vi "Psi and Delta Mapping_V2.3_RCE P=0_A_45_stokes vector.vi"() -> ()   [LabVIEW 2022 SP3]
uses:
  <vilib>/Math Plots/3D Math Plots/3D Surface/3D Surface XCtrl/3D Surface.xctl
  <vilib>/Analysis/baseanly.llb/Real A x B.vi
  <vilib>/Analysis/baseanly.llb/A x Vector.vi
  <vilib>/Utility/file.llb/Read Delimited Spreadsheet (I64).vi
  <vilib>/Analysis/baseanly.llb/Real Inverse Matrix.vi
  <vilib>/Math Plots/3D Math Plots/3D Surface/3D Surface Datatype/Public/Plot Helper (Matrix).vi
  <vilib>/Utility/file.llb/Write Delimited Spreadsheet (DBL).vi
  <vilib>/Utility/file.llb/Read Delimited Spreadsheet (DBL).vi
  <vilib>/Math Plots/3D Math Plots/3D Surface/3D Surface Datatype/3D Surface Datatype.lvclass
  <vilib>/Analysis/NI_AALBase.lvlib
panel:
  out "transposed array":dbl[][](array[numeric])
  out "x+1":i8
  in  "Tab Control":enum32{"Psi & Delta Mapping"}(tab)
  out "Drag the ROI":i64[][](graph)
  out "Location of ROI":cluster{dbl[], dbl[]}(graph)
  in  "Sampling Range (nm):":string(combo)="5"
  out "Intensity Graph 2":i64[][](graph)
  in  "Distance":dbl(slide)=1.525974025974026 scale=0.0..2.5
  in  "Map BMP File":bool
  in  "Map ASCII File":bool
  out "Psi":dbl[][](graph)
  out "Delta":dbl[][](graph)
  out "concatenated string":string
  out "concatenated string 2":string
  out "Psi Surface":refnum<class "3D Plot Datatype.lvclass">[](xcontrol)
  in  "Start (nm) :":i16=400
  in  "End (nm) :":i16=700
  in  "Save the files ?":bool
  in  "Choose an arbitrary file in the angle of incidence folder :":path
  out "Files currently reading":string
  out "Seconds":dbl
  out "Minutes":dbl
  out "Hours":dbl
  out "Delta Surface":refnum<class "3D Plot Datatype.lvclass">[](xcontrol)
  out "uniformity":cluster{i32[], dbl[]}(graph)
  out "ALL":cluster{dbl[], dbl[]}[](graph)
  in  "SE BMP & Txt File":bool
  out "Pixels :":i32(slide) scale=0.0..100.0
  in  "Psi data base":path=path "C:/Users/王家麟/Desktop/_Data/Model generate/SiO2_300nm_psi.txt"
  in  "Model index AOI25=1 ~AOI75=11":i32=4
  in  "delta data base":path=path "C:/Users/王家麟/Desktop/_Data/Model generate/SiO2_300nm_delta.txt"
  in  "Angle of Incidence :":string(combo)="55"
  out "PSI":dbl
  out "DELTA":dbl
  out "PPSI":dbl
  out "PDELTA":dbl
  out "B2":dbl
  out "a4":dbl
  out "B4":dbl
  out "XY Graph":cluster{dbl[], dbl[]}[](graph)
  in  "Psi data base 2":path=path "C:/Users/王家麟/Desktop/12.29_2D data/AOI_40_SE data_Ins_polar_285.5nm.txt"
  in  "Ins loaded":bool
  # "Wavelength Setting :"
  # "YES"
  # "NO"
  # "%"
  # "Ins index"
  # "Time spent :"
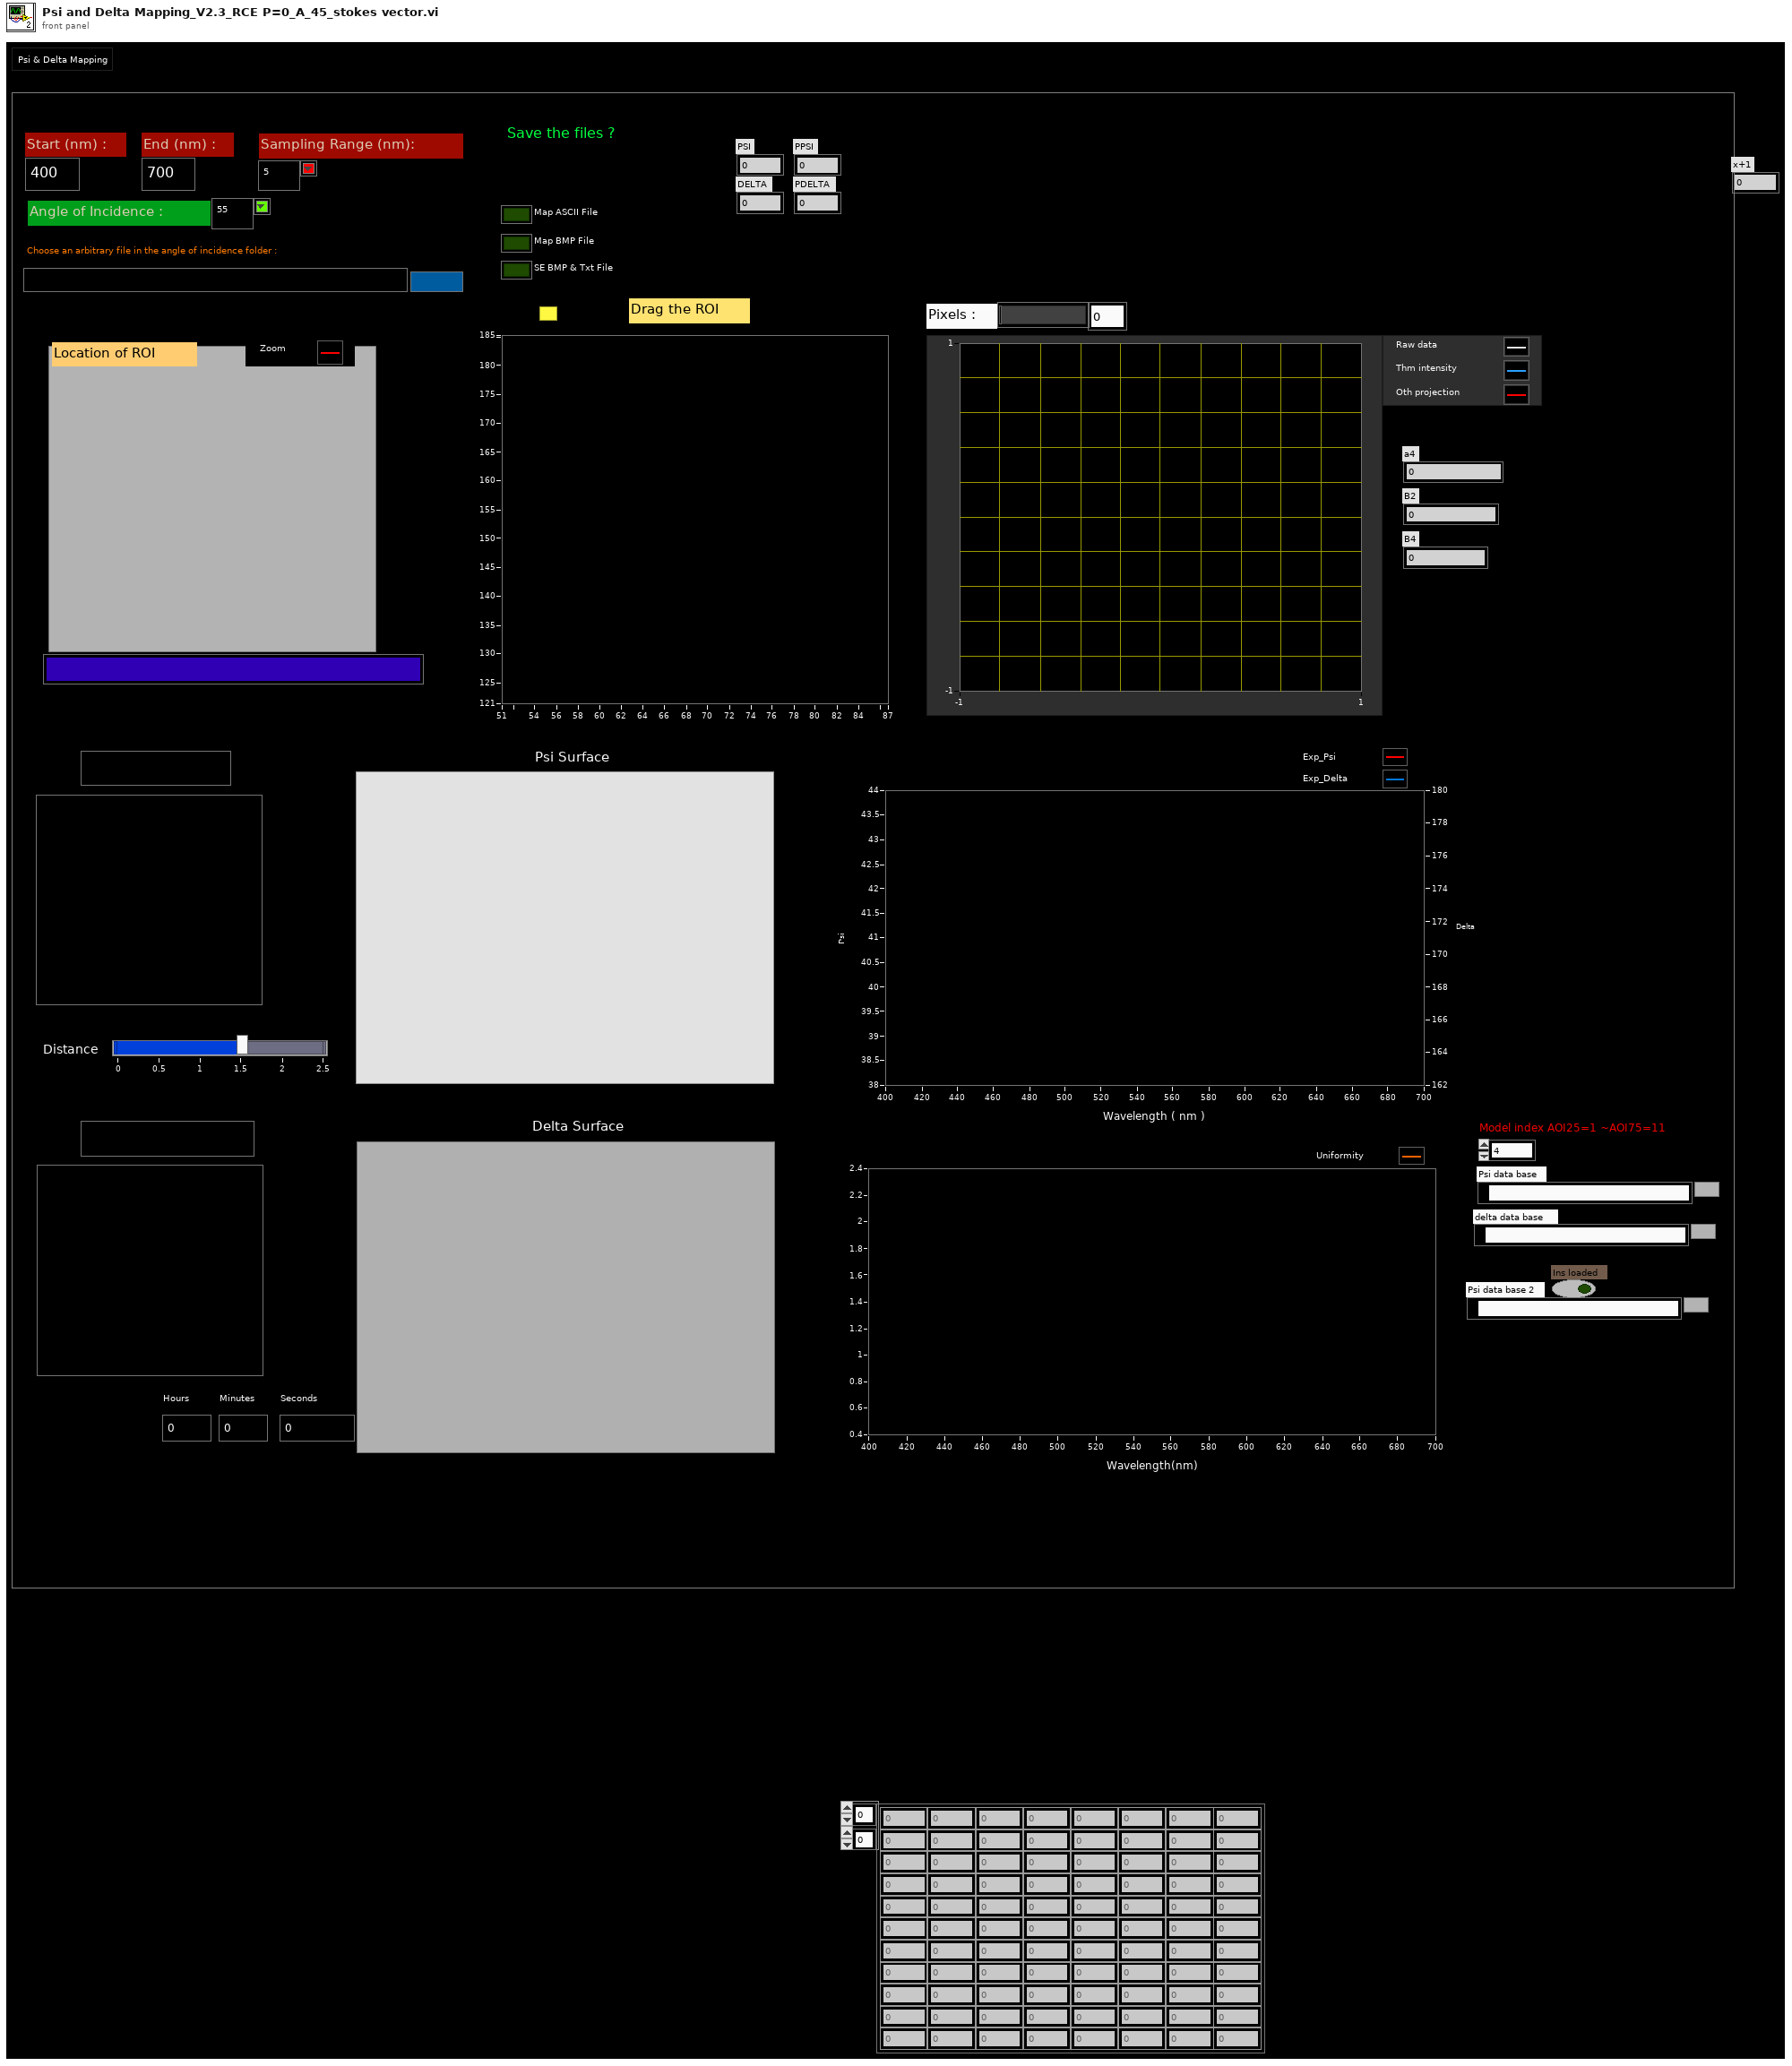
[diagram p1: front panel]
types:
  T1 = typedef "NI_Matrix.lvlib/RealMatrix.ctl" = dbl[][]
  T2 = typedef "imagedata.ctl" = cluster{"image type":i32, "image depth":i32, "image":u8[], "mask":u8[], "colors":u32[], "Rectangle":cluster{"left":i16, "top":i16, "right":i16, "bottom":i16}}
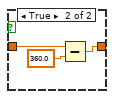
[diagram p3: hidden frame]
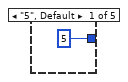
[diagram p4: hidden frame]
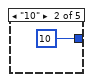
[diagram p5: hidden frame]
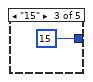
[diagram p6: hidden frame]
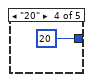
[diagram p7: hidden frame]
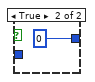
[diagram p8: hidden frame]
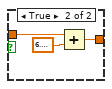
[diagram p9: hidden frame]
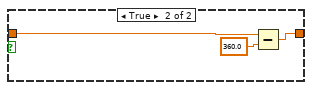
[diagram p12: hidden frame]
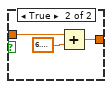
[diagram p13: hidden frame]
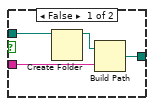
[diagram p19: hidden frame]
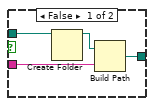
[diagram p20: hidden frame]
diagram:
  (unwired) TRUE
  (unwired) TRUE
  n1 = flat-sequence {
    tunnel: [w86] -> w8
    tunnel: [w84] -> w7
    tunnel: [w83] -> w6
    tunnel: [w21] -> w5
    tunnel: [w10] -> w4
    tunnel: [w9] -> w3
    tunnel: [w22] -> w2
    tunnel: [w20] -> w1
    tunnel: w8 -> [w681]
    tunnel: w7 -> [w680]
    tunnel: w6 -> [w679]
    tunnel: w5 -> [w678]
    tunnel: w4 -> [w677]
    tunnel: w3 -> [w676]
    tunnel: w2 -> [w675]
    tunnel: w1 -> [w674]
    frame #0 {
      w18 = u32 0 ("Plot.Y Scale Index")
      w17 = u32 1 ("Plot.Y Scale Index")
      n2 = property on="ALL" class="XYGraph (strict)"("Active Plot"=u32 0, "Plot.YScaleIdx"=w17, "Active Plot"=u32 1, "Plot.YScaleIdx"=w18, "Active Plot"=u32 2, "Plot.YScaleIdx"=w17, "Active Plot"=u32 3, "Plot.YScaleIdx"=w18, "Active Plot"=u32 4, "Plot.YScaleIdx"=w17, "Active Plot"=u32 5, "Plot.YScaleIdx"=w18, "Active Plot"=u32 6, "Plot.YScaleIdx"=w17, "Active Plot"=u32 7, "Plot.YScaleIdx"=w18) -> ()  [unwired: 2 in, 2 out]
      n3 = flat-sequence {
        tunnel: [w140] -> w62
        tunnel: "Choose an arbitrary file in the angle of incidence folder :" -> [w141]
        tunnel: w62 -> [w145]
        tunnel: [w145] -> w61
        tunnel: w61 -> [w148]
        tunnel: [w149] -> w60
        tunnel: [w150] -> w59
        tunnel: [w151] -> w58
        tunnel: [w152] -> w57
        tunnel: [w162] -> w63
        tunnel: [w163] -> w64
        tunnel: w60 -> [w158]
        tunnel: w59 -> [w163]
        tunnel: w58 -> [w159]
        tunnel: w57 -> [w162]
        tunnel: [w157] -> w56
        tunnel: [w156] -> w55
        frame #0 {
          n4 = call-poly <vilib>:"Read Delimited Spreadsheet.vi"("file path (dialog if empty)"=w141) -> ("all rows"=w140:i64[][])  [unwired: 9 in, 5 out]
        }
        frame #1 {
          w142 = 0 ("index")
          n5 = Array Size(array=w145) -> (size(s)=w147:i32[])
          n6 = Index Array(array=w147, index=w142) -> (element=w143:i32)
          n7 = Index Array(array=w147, index=1) -> (element=w144:i32)
          n8 = property on="Intensity Graph 2" class="IntGraph (strict)"("XScale.Maximum"=w143, "XScale.Minimum"=w142) -> ()  [unwired: 2 in, 2 out]
          n9 = property on="Intensity Graph 2" class="IntGraph (strict)"("YScale.Maximum"=w144, "YScale.Minimum"=w142) -> ()  [unwired: 2 in, 2 out]
        }
        frame #2 {
          "Drag the ROI" <- w148
        }
        frame #3 {
          n10 = property on="Drag the ROI" class="IntGraph (strict)"() -> ("XScale.Maximum"=w149:dbl, "XScale.Minimum"=w150:dbl)  [unwired: 2 in, 2 out]
          n11 = property on="Drag the ROI" class="IntGraph (strict)"() -> ("YScale.Maximum"=w151:dbl, "YScale.Minimum"=w152:dbl)  [unwired: 2 in, 2 out]
          n12 = Build Array(w150, w150, w149, w149, w150) -> (w155:dbl[])
          n13 = Build Array(w152, w151, w151, w152, w152) -> (w154:dbl[])
          n14 = Bundle(w155, w154) -> (→"Location of ROI":cluster{dbl[], dbl[]})  [unwired: 1 in]
        }
        frame #4 {
          n15 = Subtract(x=w158, y=w163) -> (x-y=w161:dbl)
          n16 = Subtract(x=w159, y=w162) -> (x-y=w160:dbl)
          n17 = Increment(x=w161) -> (x+1=w156:dbl)
          n18 = Increment(x=w160) -> (x+1=w157:dbl)
        }
      }
      n19 = case shown="\"25\"" "Sampling Range (nm):" {
        tunnel: [i8 5 i8 10 i8 15 i8 20 i8 25] -> w14
        frame "5", Default {
        }
        frame "10" {
        }
        frame "15" {
        }
        frame "20" {
        }
        frame "25" {
        }
      }
      n20 = Subtract(x="End (nm) :", y="Start (nm) :") -> (x-y=w70:i16)
      n21 = Divide(x=w70, y=w14) -> (x/y=w71:dbl)
      n22 = Strip Path(path="Choose an arbitrary file in the angle of incidence folder :") -> (stripped path=w28:path)  [unwired: 1 out]
      n23 = Increment(x=w71) -> (x+1=w66:dbl)
      "x+1" <- w66
      n24 = Strip Path(path=w28) -> (stripped path=w29:path)  [unwired: 1 out]
      n25 = Path To String(path=w29) -> (string=w87:string)
      n26 = for {
        N: w66 -> [_]
        tunnel: w28 -> [w172]
        tunnel: w87 -> [w201]
        tunnel: [w193] -> w73 mode=indexing
        tunnel: [w189] -> w21 mode=indexing
        tunnel: [w187] -> w74 mode=indexing
        tunnel: [w185] -> w12 mode=indexing
        tunnel: [w173] -> w84
        tunnel: [w182] -> w83
        tunnel: w14 -> [w180]
        tunnel: w56 -> [w179]
        tunnel: w55 -> [w178]
        tunnel: w63 -> [w177]
        tunnel: w64 -> [w176]
        tunnel: [w169] -> w19 mode=indexing
        i -> [w212]
        n27 = flat-sequence {
          tunnel: w212 -> [w235]
          tunnel: [w228] -> w211
          tunnel: [w227] -> w210
          tunnel: [w226] -> w209
          tunnel: [w225] -> w208
          tunnel: [w224] -> w207
          tunnel: [w223] -> w205
          tunnel: w172 -> [w213]
          tunnel: w201 -> [w222]
          tunnel: [w220] -> w190
          tunnel: [w219] -> w186
          tunnel: w180 -> [w218]
          tunnel: w179 -> [w217]
          tunnel: w178 -> [w216]
          tunnel: w177 -> [w215]
          tunnel: w176 -> [w214]
          tunnel: [w213] -> w175
          tunnel: w211 -> [w352]
          tunnel: w210 -> [w351]
          tunnel: w209 -> [w350]
          tunnel: w208 -> [w359]
          tunnel: w207 -> [w358]
          tunnel: [w356] -> w206
          tunnel: w205 -> [w356]
          tunnel: [w355] -> w202
          tunnel: [w354] -> w200
          tunnel: [w353] -> w199
          tunnel: [w346] -> w191
          tunnel: w190 -> [w346]
          tunnel: w186 -> [w342]
          tunnel: [w329] -> w184
          tunnel: w175 -> [w355]
          tunnel: [w318] -> w171
          tunnel: w206 -> [w550]
          tunnel: ["Save the files ?"] -> w204
          tunnel: [w545] -> w203
          tunnel: w202 -> [w545]
          tunnel: w200 -> [w544]
          tunnel: w199 -> [w543]
          tunnel: [w541] -> w198
          tunnel: [w542] -> w197
          tunnel: [w527] -> w196
          tunnel: [w531] -> w195
          tunnel: [w529] -> w194
          tunnel: [w528] -> w192
          tunnel: w191 -> [w528]
          tunnel: [w519] -> w188
          tunnel: w184 -> [w518]
          tunnel: [w518] -> w183
          tunnel: ["Save the files ?"] -> w182
          tunnel: ["Map BMP File"] -> w181
          tunnel: w171 -> [w514]
          tunnel: [w514] -> w170
          tunnel: w194 -> [w558]
          tunnel: w195 -> [w559]
          tunnel: w196 -> [w560]
          tunnel: w197 -> [w561]
          tunnel: w198 -> [w562]
          tunnel: w203 -> [w563]
          tunnel: w204 -> [w564]
          tunnel: [w558] -> w193
          tunnel: [w557] -> w189
          tunnel: w192 -> [w557]
          tunnel: [w556] -> w187
          tunnel: w188 -> [w556]
          tunnel: [w555] -> w185
          tunnel: w183 -> [w555]
          tunnel: [w554] -> w174
          tunnel: w181 -> [w553]
          tunnel: w170 -> [w552]
          tunnel: [w552] -> w169
          frame #0 {
            n28 = Multiply(x=w235, y=w218) -> (x*y=w237:i32)
            n29 = local read "Start (nm) :"() -> (w236:i16)
            n30 = Add(x=w236, y=w237) -> (x+y=w220:i32)
            n31 = Number To Decimal String(number=w220) -> (decimal integer string=w223:string)  [unwired: 1 in]
            n32 = Concatenate Strings(w222, "\\" ("string"), w223, "nm\\" ("string")) -> (w233:string)
            n33 = for {
              N: i8 15 -> [_]
              tunnel: w233 -> [w260]
              tunnel: w223 -> [w259]
              tunnel: [w258] -> w228 mode=indexing
              tunnel: [w256] -> w225
              tunnel: [w255] -> w224
              tunnel: [w257] -> w219 mode=indexing
              tunnel: w217 -> [w254]
              tunnel: w216 -> [w253]
              tunnel: w215 -> [w252]
              tunnel: w214 -> [w251]
              i -> [w263]
              n34 = Increment(x=w263) -> (x+1=w262:i32)
              n35 = Number To Decimal String(number=w262) -> (decimal integer string=w266:string)  [unwired: 1 in]
              n36 = Concatenate Strings(w260, w259, " (" ("string"), w266, ").asc" ("string")) -> (w265:string)
              n37 = String To Path(string=w265) -> (path=w250:path)
              n38 = flat-sequence {
                tunnel: w250 -> [w275]
                tunnel: w251 -> [w276]
                tunnel: w252 -> [w277]
                tunnel: w253 -> [w278]
                tunnel: w254 -> [w279]
                tunnel: [w279] -> w242
                tunnel: [w278] -> w241
                tunnel: [w277] -> w240
                tunnel: [w276] -> w239
                tunnel: [w267] -> w238
                tunnel: [w295] -> w249
                tunnel: [w289] -> w248
                tunnel: [w288] -> w247
                tunnel: [w292] -> w246
                tunnel: [w288] -> w245
                tunnel: [w290] -> w244
                tunnel: [w291] -> w243
                tunnel: w238 -> [w280]
                tunnel: w239 -> [w284]
                tunnel: w240 -> [w285]
                tunnel: w241 -> [w286]
                tunnel: w242 -> [w287]
                tunnel: [w301] -> w255
                tunnel: [w302] -> w256
                tunnel: [w303] -> w257
                tunnel: [w296] -> w258
                tunnel: w249 -> [w303]
                tunnel: w248 -> [w302]
                tunnel: w247 -> [w301]
                tunnel: w246 -> [w300]
                tunnel: w245 -> [w299]
                tunnel: w244 -> [w298]
                tunnel: w243 -> [w297]
                frame #0 {
                  n39 = call-poly <vilib>:"Read Delimited Spreadsheet.vi"("file path (dialog if empty)"=w275) -> ("new file path (Not A Path if cancelled)"=w274:path, "all rows"=w267:i64[][])  [unwired: 9 in, 4 out]
                  "Intensity Graph 2" <- w267
                  n40 = Strip Path(path=w274) -> (stripped path=w273:path, name=w270:string)
                  n41 = Strip Path(path=w273) -> (name=w272:string)  [unwired: 1 out]
                  n42 = Concatenate Strings("Files currently reading : " ("string"), w272, "\\" ("string"), w270) -> (→"Files currently reading":string)
                }
                frame #1 {
                  w291 = 75 ("Dark counts")
                  n43 = Array Subset(array=w280, index (row)=w284, length (row)=w286, index (col)=w285, length (col)=w287) -> (w290:i64[][])
                  n44 = local write "Drag the ROI"(w280) -> ()
                  n45 = Add Array Elements(numeric array=w290) -> (sum=w294:i64)
                  n46 = Array Size(array=w290) -> (size(s)=w283:i32[])
                  n47 = Index Array(array=w283, index=1) -> (element=w289:i32)
                  n48 = Index Array(array=w283, index=0) -> (element=w288:i32)
                  n49 = Multiply(x=w289, y=w288) -> (x*y=w292:i32)
                  n50 = Multiply(x=w292, y=w291) -> (x*y=w293:i32)
                  n51 = Subtract(x=w294, y=w293) -> (x-y=w295:i64)
                }
                frame #2 {
                  n52 = for {
                    N: w300 -> [_]
                    tunnel: w299 -> [w312]
                    tunnel: w298 -> [w304]
                    tunnel: [w307] -> w296 mode=indexing
                    tunnel: w297 -> [w306]
                    i -> [w313]
                    n53 = Quotient & Remainder(x=w313, y=w312) -> (x-y*floor(x/y)=w311:i32, floor(x/y)=w310:i32)
                    n54 = Index Array(array=w304, index (row)=w311, index (col)=w310) -> (element=w305:i64)
                    n55 = Subtract(x=w305, y=w306) -> (x-y=w308:i64)
                    n56 = Less Than 0?(x=w308) -> (x < 0?=w309:bool)
                    n57 = case shown="False" w309 {
                      tunnel: [w314 i8 0] -> w307
                      tunnel: w308 -> [w314 _]
                      frame False {
                      }
                      frame True {
                      }
                    }
                  }
                }
              }
            }
            n58 = Array Size(array=w228) -> (size(s)=w229:i32[])
            n59 = Index Array(array=w229, index=1) -> (element=w226:i32)
            n60 = Index Array(array=w229, index=0) -> (element=w227:i32)
          }
          frame #1 {
            w357 = 0.0
            n61 = property on="Delta" class="IntGraph (strict)"("YScale.Maximum"=w359, "YScale.Minimum"=w357) -> ()  [unwired: 2 in, 2 out]
            n62 = for {
              N: i8 15 -> [_]
              tunnel: [w383] -> w340 mode=indexing
              tunnel: [w382] -> w341 mode=indexing
              i -> [w386]
              n63 = Increment(x=w386) -> (x+1=w385:i32)
              n64 = Multiply(x=24.0, y=w385) -> (x*y=w382:dbl)
              n65 = expression code="(x/180.0)*pi" "degrees to radians"(w382) -> (w381:dbl)
              n66 = formula code="float c1,c2,c3,c4;\nc1=1;\nc2=sin(2*C);\nc3=cos(4*C);\nc4=sin(4*C);"("C"=w381) -> ("c2"=w380:dbl, "c3"=w379:dbl, "c4"=w378:dbl, "c1"=w377:dbl)
              n67 = Build Array(w377, w380, w379, w378) -> (w383:dbl[])
            }
            n68 = property on="Psi" class="IntGraph (strict)"("YScale.Maximum"=w359, "YScale.Minimum"=w357) -> ()  [unwired: 2 in, 2 out]
            n69 = property on="Psi" class="IntGraph (strict)"("XScale.Maximum"=w358, "XScale.Minimum"=w357) -> ()  [unwired: 2 in, 2 out]
            n70 = property on="Delta" class="IntGraph (strict)"("XScale.Maximum"=w358, "XScale.Minimum"=w357) -> ()  [unwired: 2 in, 2 out]
            n71 = Transpose 2D Array(2D array=w340) -> (transposed array=w339:dbl[][])
            n72 = for {
              N: w350 -> [w458]
              tunnel: w352 -> [w464]
              tunnel: w351 -> [w461]
              tunnel: [w387] -> w349 mode=indexing
              tunnel: [w443] -> w348 mode=indexing
              tunnel: w340 -> [w451]
              tunnel: w341 -> [w435]
              i -> [w460]
              n73 = Transpose 2D Array(2D array=w451) -> (transposed array=w450:dbl[][])
              n74 = call-poly <vilib>:"A x B.vi"("B"=w451, "A"=w450) -> ("A x B"=w454:T1)  [unwired: 1 out]
              n75 = Increment(x=w460) -> (x+1=w459:i32)
              n76 = Array Subset(array=w464, index (col)=w460, length (col)=1 ("length")) -> (w462:i64[][])  [unwired: 2 in]
              n77 = Divide(x=w459, y=w458) -> (x/y=w457:dbl)
              n78 = call-poly <vilib>:"Inverse Matrix.vi"("Input Matrix"=w454) -> ("Inverse Matrix"=w453:T1)  [unwired: 1 in, 1 out]
              n79 = Reshape Array(w462, w461) -> (w422:i64[])
              n80 = call-poly <vilib>:"A x B.vi"("B"=w450, "A"=w453) -> ("A x B"=w452:T1)  [unwired: 1 out]
              n81 = Array Max & Min(array=w422) -> (max value=w423:i64)  [unwired: 3 out]
              n82 = Multiply(x=i8 100, y=w457) -> (x*y=→"Pixels :":dbl)
              n83 = Divide(x=w422, y=w423) -> (x/y=w421:dbl[])
              n84 = call-poly <vilib>:"A x B.vi"("Vector"=w422, "A"=w452) -> ("A x Vector"=w449:dbl[])  [unwired: 1 out]
              n85 = call-poly <vilib>:"A x B.vi"("Vector"=w449, "A"=w451) -> ("A x Vector"=w416:dbl[])  [unwired: 1 out]
              n86 = Index Array(array=w449, index #1=0 ("index"), index #2=1 ("index"), index #3=2 ("index"), index #4=3 ("index")) -> (element #1=w425:dbl, element #2=w434:dbl, element #3=w444:dbl, element #4=w433:dbl)
              n87 = Array Max & Min(array=w416) -> (max value=w417:dbl)  [unwired: 3 out]
              n88 = formula code="float psi, delta ;\n\npsi = 0.5*atan(sqrt((0.5*B2)**2+\n                           (B4)**2)/(-a4)) ;\ndelta = atan(0.5*B2/B4) ;\nx=sign(B2);\ny=sign(B4);"("B2"=w434, "a4"=w444, "B4"=w433, "r"=w425) -> ("psi"=w441:dbl, "delta"=w427:dbl, "x"=w426:dbl, "y"=w428:dbl)
              n89 = Divide(x=w416, y=w417) -> (x/y=w415:dbl[])
              n90 = Greater Than 0?(x=w426) -> (x > 0?=w432:bool)
              n91 = Greater Than 0?(x=w428) -> (x > 0?=w430:bool)
              n92 = Less Than 0?(x=w441) -> (x < 0?=w442:bool)
              n93 = And(x=w432, y=w430) -> (x .and. y?=w431:bool)
              n94 = case shown="True" w442 {
                tunnel: w441 -> [w494 w497]
                tunnel: [w494 w496] -> w440
                frame False {
                }
                frame True {
                  n95 = Add(x=w497, y=1.5707963267948966) -> (x+y=w496:dbl)
                }
              }
              n96 = case shown="False" w431 {
                tunnel: w427 -> [w486 w493]
                tunnel: [w484 w493] -> w429
                tunnel: w426 -> [w485 _]
                tunnel: w430 -> [w481 _]
                frame False {
                  n97 = Less Than 0?(x=w485) -> (x < 0?=w483:bool)
                  n98 = And(x=w481, y=w483) -> (x .and. y?=w482:bool)
                  n99 = case shown="False" w482 {
                    tunnel: w486 -> [w487 w491]
                    tunnel: [w488 w490] -> w484
                    frame False {
                      n100 = Add(x=w487, y=3.141592653589793) -> (x+y=w488:dbl)
                    }
                    frame True {
                      n101 = Add(x=w491, y=6.283185307179586) -> (x+y=w490:dbl)
                    }
                  }
                }
                frame True {
                }
              }
              n102 = expression code="(x/pi)*180.0" "radians to degrees"(w440) -> (w443:dbl)
              "PPSI" <- w443
              n103 = expression code="(x/pi)*180.0" "radians to degrees"(w429) -> (w388:dbl)
              n104 = for {
                tunnel: w425 -> [w503]
                tunnel: [w502] -> w419 mode=indexing
                tunnel: w435 -> [w501] mode=indexing
                tunnel: w440 -> [w499]
                tunnel: w429 -> [w500]
                tunnel: [w498] -> w424 mode=indexing
                n105 = expression code="(x/180.0)*pi" "degrees to radians"(w501) -> (w498:dbl)
                n106 = formula code="float S1,S2 ,S3;\n\nS1 = - cos(2*a);\nS2 =  sin(2*a)*cos(b);\nS3 = -sin(2*a)*sin(b);\nI = r * (1+0.577*S1*cos(4*C)\n           -S3*sin(2*C)\n            +0.5*S2*sin(4*C)) ;"("r"=w503, "a"=w499, "b"=w500, "C"=w498) -> ("I"=w502:dbl)
              }
              n107 = Greater?(x=w388, y=360.0) -> (0:w390:bool)
              n108 = case shown="False" w390 {
                tunnel: w388 -> [w465 w467]
                tunnel: [w465 w466] -> w387
                frame False {
                }
                frame True {
                  n109 = Subtract(x=w467, y=360.0) -> (x-y=w466:dbl)
                }
              }
              "PDELTA" <- w387
              n110 = for {
                tunnel: w421 -> [w480] mode=indexing
                tunnel: w424 -> [w479] mode=indexing
                tunnel: [w478] -> w412 mode=indexing
                tunnel: [w477] -> w400 mode=indexing
                n111 = formula code="float x,y;\nx=I*cos(p);\ny=I*sin(p);"("I"=w480, "p"=w479) -> ("x"=w478:dbl, "y"=w477:dbl)
              }
              n112 = Array Max & Min(array=w419) -> (max value=w420:dbl)  [unwired: 3 out]
              n113 = for {
                tunnel: w415 -> [w472] mode=indexing
                tunnel: w424 -> [w471] mode=indexing
                tunnel: [w470] -> w404 mode=indexing
                tunnel: [w469] -> w392 mode=indexing
                n114 = formula code="float x,y;\nx=I*cos(p);\ny=I*sin(p);"("I"=w472, "p"=w471) -> ("x"=w470:dbl, "y"=w469:dbl)
              }
              n115 = Divide(x=w419, y=w420) -> (x/y=w418:dbl[])
              n116 = for {
                tunnel: w418 -> [w476] mode=indexing
                tunnel: w424 -> [w475] mode=indexing
                tunnel: [w474] -> w408 mode=indexing
                tunnel: [w473] -> w396 mode=indexing
                n117 = formula code="float x,y;\nx=I*cos(p);\ny=I*sin(p);"("I"=w476, "p"=w475) -> ("x"=w474:dbl, "y"=w473:dbl)
              }
              n118 = Index Array(array=w412, index=0) -> (element=w413:dbl)
              n119 = Index Array(array=w400, index=0) -> (element=w401:dbl)
              n120 = Index Array(array=w404, index=0) -> (element=w405:dbl)
              n121 = Index Array(array=w392, index=0) -> (element=w393:dbl)
              n122 = Build Array (concatenate)(w412, w413) -> (w411:dbl[])
              n123 = Build Array (concatenate)(w400, w401) -> (w399:dbl[])
              n124 = Build Array (concatenate)(w404, w405) -> (w403:dbl[])
              n125 = Build Array (concatenate)(w392, w393) -> (w391:dbl[])
              n126 = Index Array(array=w408, index=0) -> (element=w409:dbl)
              n127 = Index Array(array=w396, index=0) -> (element=w397:dbl)
              n128 = Build Array (concatenate)(w408, w409) -> (w407:dbl[])
              n129 = Build Array (concatenate)(w396, w397) -> (w395:dbl[])
              n130 = Bundle(w403, w391) -> (w436:cluster{dbl[], dbl[]})  [unwired: 1 in]
              n131 = Bundle(w411, w399) -> (w439:cluster{dbl[], dbl[]})  [unwired: 1 in]
              n132 = Bundle(w407, w395) -> (w437:cluster{dbl[], dbl[]})  [unwired: 1 in]
              n133 = Build Array(w439, w437, w436) -> (→"XY Graph":cluster{dbl[], dbl[]}[])
            }
            n134 = call-poly <vilib>:"A x B.vi"("B"=w340, "A"=w339) -> ("A x B"=w345:T1)  [unwired: 1 out]
            n135 = call-poly <vilib>:"Inverse Matrix.vi"("Input Matrix"=w345) -> ("Inverse Matrix"=w344:T1)  [unwired: 1 in, 1 out]
            n136 = call-poly <vilib>:"A x B.vi"("B"=w339, "A"=w344) -> ("A x B"=w343:T1)  [unwired: 1 out]
            n137 = call-poly <vilib>:"A x B.vi"("Vector"=w342, "A"=w343) -> ("A x Vector"=w334:dbl[])  [unwired: 1 out]
            n138 = Index Array(array=w334, index #1=0 ("index"), index #2=1 ("index"), index #3=2 ("index"), index #4=3 ("index")) -> (element #1=w319:dbl, element #2=w328:dbl, element #3=w333:dbl, element #4=w327:dbl)
            "B2" <- w328
            "a4" <- w333
            "B4" <- w327
            n139 = formula code="float psi, delta ;\n\npsi = 0.5*atan(sqrt((0.5*B2)**2+\n                           (B4)**2)/(-a4)) ;\ndelta = atan(0.5*B2/B4) ;\nx=sign(B2);\ny=sign(B4);"("B2"=w328, "a4"=w333, "B4"=w327, "r"=w319) -> ("psi"=w330:dbl, "delta"=w323:dbl, "x"=w322:dbl, "y"=w326:dbl)
            n140 = Less Than 0?(x=w330) -> (x < 0?=w332:bool)
            n141 = Greater Than 0?(x=w322) -> (x > 0?=w325:bool)
            n142 = Greater Than 0?(x=w326) -> (x > 0?=w320:bool)
            n143 = And(x=w325, y=w320) -> (x .and. y?=w324:bool)
            n144 = case shown="True" w332 {
              tunnel: w330 -> [w373 w376]
              tunnel: [w373 w375] -> w331
              frame False {
              }
              frame True {
                n145 = Add(x=w376, y=1.5707963267948966) -> (x+y=w375:dbl)
              }
            }
            n146 = case shown="False" w324 {
              tunnel: w323 -> [w365 w372]
              tunnel: [w363 w372] -> w321
              tunnel: w322 -> [w364 _]
              tunnel: w320 -> [w360 _]
              frame False {
                n147 = Less Than 0?(x=w364) -> (x < 0?=w362:bool)
                n148 = And(x=w360, y=w362) -> (x .and. y?=w361:bool)
                n149 = case shown="False" w361 {
                  tunnel: w365 -> [w366 w370]
                  tunnel: [w367 w369] -> w363
                  frame False {
                    n150 = Add(x=w366, y=3.141592653589793) -> (x+y=w367:dbl)
                  }
                  frame True {
                    n151 = Add(x=w370, y=6.283185307179586) -> (x+y=w369:dbl)
                  }
                }
              }
              frame True {
              }
            }
            n152 = expression code="(x/pi)*180.0" "radians to degrees"(w331) -> (w317:dbl)
            "PSI" <- w317
            n153 = Add(x=w317, y=0.0) -> (x+y=w318:dbl)
            n154 = expression code="(x/pi)*180.0" "radians to degrees"(w321) -> (w329:dbl)
            "DELTA" <- w329
            n155 = for {
              N: w359 -> [_]
              tunnel: w349 -> [w512]
              tunnel: w358 -> [w510]
              tunnel: [w509] -> w354 mode=indexing
              i -> [w511]
              n156 = Multiply(x=w510, y=w511) -> (x*y=w513:i32)
              n157 = Array Subset(array=w512, index=w513, length=w510) -> (w509:dbl[])
            }
            n158 = for {
              N: w359 -> [_]
              tunnel: w348 -> [w508]
              tunnel: w358 -> [w505]
              tunnel: [w504] -> w353 mode=indexing
              i -> [w507]
              n159 = Multiply(x=w505, y=w507) -> (x*y=w506:i32)
              n160 = Array Subset(array=w508, index=w506, length=w505) -> (w504:dbl[])
            }
          }
          frame #2 {
            # "Delta"
            # "PSI"
            n161 = Transpose 2D Array(2D array=w544) -> (transposed array=w527:dbl[][])
            "Delta" <- w527
            n162 = Concatenate Strings("Psi_" ("string"), w550, "nm" ("string")) -> (w541:string)
            "concatenated string" <- w541
            n163 = property on="Psi Surface" class="3D Surface (strict)"("Graph: View Distance"="Distance") -> ()  [unwired: 2 in, 2 out]
            n164 = property on="Delta Surface" class="3D Surface (strict)"("Graph: View Distance"="Distance") -> ()  [unwired: 2 in, 2 out]
            n165 = Transpose 2D Array(2D array=w543) -> (transposed array=w531:dbl[][])
            "Psi" <- w531
            n166 = Concatenate Strings("Delta_" ("string"), w550, "nm" ("string")) -> (w542:string)
            "concatenated string 2" <- w542
            n167 = Add Array Elements(numeric array=w527) -> (sum=w520:dbl)
            n168 = And(x="Map BMP File", y="Save the files ?") -> (x .and. y?=w515:bool)
            n169 = call-poly <vilib>:"Plot Helper.vi"("z matrix"=w527) -> ("3D Plot lvclass Array out"=→"Delta Surface":refnum<class "3D Plot Datatype.lvclass">[])  [unwired: 5 in, 5 out]
            n170 = Array Size(array=w527) -> (size(s)=w524:i32[])
            n171 = case shown="True" w515 {
              frame False {
              }
              frame True {
                n172 = Wait (ms)(milliseconds to wait=u32 800) -> ()  [unwired: 1 out]
              }
            }
            n173 = Add Array Elements(numeric array=w531) -> (sum=w530:dbl)
            n174 = call-poly <vilib>:"Plot Helper.vi"("z matrix"=w531) -> ("3D Plot lvclass Array out"=→"Psi Surface":refnum<class "3D Plot Datatype.lvclass">[])  [unwired: 5 in, 5 out]
            n175 = Index Array(array=w524, index=0) -> (element=w523:i32)
            n176 = Index Array(array=w524, index=1) -> (element=w522:i32)
            n177 = Array Size(array=w531) -> (size(s)=w536:i32[])
            n178 = Multiply(x=w523, y=w522) -> (x*y=w521:i32)
            n179 = Index Array(array=w536, index=0) -> (element=w534:i32)
            n180 = Index Array(array=w536, index=1) -> (element=w533:i32)
            n181 = Multiply(x=w534, y=w533) -> (x*y=w532:i32)
            n182 = Divide(x=w520, y=w521) -> (x/y=w519:dbl)
            n183 = Divide(x=w530, y=w532) -> (x/y=w529:dbl)
          }
          frame #3 {
            n184 = case shown="True" w564 {
              tunnel: w563 -> [_ w566]
              tunnel: w562 -> [_ w567]
              tunnel: w561 -> [_ w568]
              tunnel: w560 -> [_ w570]
              tunnel: w559 -> [_ w569]
              tunnel: [_ w567] -> _
              tunnel: [_ w566] -> w554
              tunnel: w553 -> [_ w565]
              frame False {
              }
              frame True {
                n185 = case shown="True" w565 {
                  tunnel: w568 -> [_ w578]
                  tunnel: w567 -> [_ w585]
                  tunnel: w566 -> [_ w591]
                  frame False {
                  }
                  frame True {
                    w592 = 24 ("Image Depth")
                    n186 = Strip Path(path=w591) -> (stripped path=w579:path)  [unwired: 1 out]
                    n187 = Build Path(base path=w579, name or relative path="BMP_Psi") -> (appended path=w586:path)
                    n188 = Build Path(base path=w579, name or relative path="BMP_Delta") -> (appended path=w580:path)
                    n189 = call <vilib>:"Check if File or Folder Exists.vi"("path"=w586) -> ("file or folder exists?"=w587:bool, "dup path"=w588:path)  [unwired: 8 in, 1 out]
                    n190 = call <vilib>:"Check if File or Folder Exists.vi"("path"=w580) -> ("file or folder exists?"=w581:bool, "dup path"=w582:path)  [unwired: 8 in, 1 out]
                    n191 = case shown="True" w587 {
                      tunnel: w588 -> [w619 w622]
                      tunnel: [w618 w621] -> w589
                      tunnel: w585 -> [w616 w620]
                      frame False {
                        n192 = Create Folder(path (use dialog)=w619) -> (created path=w617:path)  [unwired: 2 in, 2 out]
                        n193 = Build Path(base path=w617, name or relative path=w616) -> (appended path=w618:path)
                      }
                      frame True {
                        n194 = Build Path(base path=w622, name or relative path=w620) -> (appended path=w621:path)
                      }
                    }
                    n195 = case shown="True" w581 {
                      tunnel: w582 -> [w612 w615]
                      tunnel: [w611 w614] -> w583
                      tunnel: w578 -> [w609 w613]
                      frame False {
                        n196 = Create Folder(path (use dialog)=w612) -> (created path=w610:path)  [unwired: 2 in, 2 out]
                        n197 = Build Path(base path=w610, name or relative path=w609) -> (appended path=w611:path)
                      }
                      frame True {
                        n198 = Build Path(base path=w615, name or relative path=w613) -> (appended path=w614:path)
                      }
                    }
                    n199 = Path To String(path=w589) -> (string=w584:string)
                    n200 = Path To String(path=w583) -> (string=w577:string)
                    n201 = Concatenate Strings(w585, ".bmp" ("string")) -> (w607:string)
                    n202 = Concatenate Strings(w578, ".bmp" ("string")) -> (w608:string)
                    n203 = Concatenate Strings(w584, w607) -> (w603:string)
                    n204 = Concatenate Strings(w577, w608) -> (w604:string)
                    n205 = invoke on="Psi Surface" class="3D Surface (strict)" method="Get Image"("image depth"=w592) -> ("image data"=w601:T2)  [unwired: 5 in, 5 out]
                    n206 = invoke on="Delta Surface" class="3D Surface (strict)" method="Get Image"("image depth"=w592) -> ("image data"=w602:T2)  [unwired: 5 in, 5 out]
                    n207 = String To Path(string=w603) -> (path=w605:path)
                    n208 = String To Path(string=w604) -> (path=w606:path)
                    n209 = call <vilib>:"Write BMP File.vi"("image data"=w601, "path to BMP file"=w605) -> ("path"=w574:path)  [unwired: 8 in, 1 out]
                    n210 = call <vilib>:"Write BMP File.vi"("image data"=w602, "path to BMP file"=w606) -> ("path"=w572:path)  [unwired: 8 in, 1 out]
                    n211 = Strip Path(path=w574) -> (stripped path=w598:path)  [unwired: 1 out]
                    n212 = Strip Path(path=w572) -> (stripped path=w600:path)  [unwired: 1 out]
                    n213 = Build Path(base path=w598, name or relative path=w607) -> (appended path=w597:path)
                    n214 = Build Path(base path=w600, name or relative path=w608) -> (appended path=w599:path)
                    n215 = Copy(9:TRUE ("overwrite (F)"), 10:w597, 11:w574) -> (0:w575:errorcluster)  [unwired: 2 in, 2 out]
                    n216 = Copy(9:TRUE ("overwrite (F)"), 10:w599, 11:w572) -> (0:w573:errorcluster)  [unwired: 2 in, 2 out]
                    n217 = Delete(path (use dialog)=w574, error in=w575) -> ()  [unwired: 3 in, 3 out]
                    n218 = Delete(path (use dialog)=w572, error in=w573) -> ()  [unwired: 3 in, 3 out]
                  }
                }
                n219 = case shown="True" "Map ASCII File" {
                  tunnel: w568 -> [_ w624]
                  tunnel: w567 -> [_ w623]
                  tunnel: w570 -> [_ w646]
                  tunnel: w569 -> [_ w640]
                  tunnel: w566 -> [_ w634]
                  frame False {
                  }
                  frame True {
                    w649 = ".txt" ("string")
                    n220 = Strip Path(path=w634) -> (stripped path=w626:path)  [unwired: 1 out]
                    n221 = Concatenate Strings(w623, w649) -> (w658:string)
                    n222 = Concatenate Strings(w624, w649) -> (w659:string)
                    n223 = Build Path(base path=w626, name or relative path="ASCII_Psi") -> (appended path=w635:path)
                    n224 = Build Path(base path=w626, name or relative path="ASCII_Delta") -> (appended path=w628:path)
                    n225 = call <vilib>:"Check if File or Folder Exists.vi"("path"=w635) -> ("file or folder exists?"=w636:bool, "dup path"=w637:path)  [unwired: 8 in, 1 out]
                    n226 = call <vilib>:"Check if File or Folder Exists.vi"("path"=w628) -> ("file or folder exists?"=w629:bool, "dup path"=w630:path)  [unwired: 8 in, 1 out]
                    n227 = case shown="True" w636 {
                      tunnel: w637 -> [w670 w673]
                      tunnel: [w669 w672] -> w638
                      tunnel: w623 -> [w667 w671]
                      frame False {
                        n228 = Create Folder(path (use dialog)=w670) -> (created path=w668:path)  [unwired: 2 in, 2 out]
                        n229 = Build Path(base path=w668, name or relative path=w667) -> (appended path=w669:path)
                      }
                      frame True {
                        n230 = Build Path(base path=w673, name or relative path=w671) -> (appended path=w672:path)
                      }
                    }
                    n231 = case shown="True" w629 {
                      tunnel: w630 -> [w663 w666]
                      tunnel: [w662 w665] -> w631
                      tunnel: w624 -> [w660 w664]
                      frame False {
                        n232 = Create Folder(path (use dialog)=w663) -> (created path=w661:path)  [unwired: 2 in, 2 out]
                        n233 = Build Path(base path=w661, name or relative path=w660) -> (appended path=w662:path)
                      }
                      frame True {
                        n234 = Build Path(base path=w666, name or relative path=w664) -> (appended path=w665:path)
                      }
                    }
                    n235 = Path To String(path=w638) -> (string=w632:string)
                    n236 = Path To String(path=w631) -> (string=w625:string)
                    n237 = Concatenate Strings(w632, w623) -> (w656:string)
                    n238 = Concatenate Strings(w625, w624) -> (w657:string)
                    n239 = String To Path(string=w656) -> (path=w641:path)
                    n240 = String To Path(string=w657) -> (path=w643:path)
                    n241 = call-poly <vilib>:"Write Delimited Spreadsheet.vi"("file path (dialog if empty)"=w641, "2D data"=w640, "append to file? (new file:F)"=FALSE) -> ("new file path (Not A Path if cancelled)"=w642:path)  [unwired: 11 in, 1 out]
                    n242 = call-poly <vilib>:"Write Delimited Spreadsheet.vi"("file path (dialog if empty)"=w643, "2D data"=w646, "append to file? (new file:F)"=FALSE) -> ("new file path (Not A Path if cancelled)"=w644:path)  [unwired: 11 in, 1 out]
                    n243 = Strip Path(path=w642) -> (stripped path=w651:path)  [unwired: 1 out]
                    n244 = Strip Path(path=w644) -> (stripped path=w654:path)  [unwired: 1 out]
                    n245 = Build Path(base path=w651, name or relative path=w658) -> (appended path=w650:path)
                    n246 = Build Path(base path=w654, name or relative path=w659) -> (appended path=w653:path)
                    n247 = Copy(9:TRUE ("overwrite (F)"), 10:w650, 11:w642) -> (0:w652:errorcluster)  [unwired: 2 in, 2 out]
                    n248 = Copy(9:TRUE ("overwrite (F)"), 10:w653, 11:w644) -> (0:w655:errorcluster)  [unwired: 2 in, 2 out]
                    n249 = Delete(path (use dialog)=w642, error in=w652) -> ()  [unwired: 3 in, 3 out]
                    n250 = Delete(path (use dialog)=w644, error in=w655) -> ()  [unwired: 3 in, 3 out]
                  }
                }
              }
            }
          }
        }
        n251 = Strip Path(path=w174) -> (stripped path=w173:path)  [unwired: 1 out]
      }
      n252 = call-poly <vilib>:"Read Delimited Spreadsheet.vi"("file path (dialog if empty)"="Psi data base") -> ("all rows"=w53:dbl[][])  [unwired: 9 in, 5 out]
      n253 = call-poly <vilib>:"Read Delimited Spreadsheet.vi"("file path (dialog if empty)"="delta data base") -> ("all rows"=w37:dbl[][])  [unwired: 9 in, 5 out]
      n254 = Array Subset(array=w53, index (col)="Model index AOI25=1 ~AOI75=11", length (col)=1 ("length")) -> (w49:dbl[][])  [unwired: 2 in]
      n255 = Array Subset(array=w37, index (col)="Model index AOI25=1 ~AOI75=11", length (col)=1 ("length")) -> (w45:dbl[][])  [unwired: 2 in]
      n256 = Array Size(array=w49) -> (size(s)=w51:i32[])
      n257 = Array Size(array=w45) -> (size(s)=w47:i32[])
      n258 = Array Max & Min(array=w51) -> (max value=w50:i32)  [unwired: 3 out]
      n259 = Array Max & Min(array=w47) -> (max value=w46:i32)  [unwired: 3 out]
      n260 = Reshape Array(w49, w50) -> (w27:dbl[])
      n261 = Reshape Array(w45, w46) -> (w26:dbl[])
      n262 = Subtract(x=w74, y=w12) -> (x-y=w80:dbl[])
      n263 = Subtract(x=w73, y=w19) -> (x-y=w79:dbl[])
      n264 = for {
        tunnel: w27 -> [w135] mode=indexing
        tunnel: w26 -> [w133] mode=indexing
        tunnel: w19 -> [w139] mode=indexing
        tunnel: w12 -> [w137] mode=indexing
        tunnel: [w130] -> w20 mode=indexing
        tunnel: [w128] -> w22 mode=indexing
        n265 = expression code="(x/180.0)*pi" "degrees to radians"(w139) -> (w138:dbl)
        n266 = expression code="(x/180.0)*pi" "degrees to radians"(w137) -> (w136:dbl)
        n267 = expression code="(x/180.0)*pi" "degrees to radians"(w135) -> (w134:dbl)
        n268 = expression code="(x/180.0)*pi" "degrees to radians"(w133) -> (w132:dbl)
        n269 = formula code="float p3,d3;\np3=atan(tan(p1)\n          /tan(p2));\nd3=d1-d2;"("p2"=w134, "d2"=w132, "p1"=w138, "d1"=w136) -> ("p3"=w131:dbl, "d3"=w129:dbl)
        n270 = expression code="(x/pi)*180.0" "radians to degrees"(w131) -> (w130:dbl)
        n271 = expression code="(x/pi)*180.0" "radians to degrees"(w129) -> (w128:dbl)
      }
      n272 = Square(x=w80) -> (x^2=w78:dbl[])
      n273 = Square(x=w79) -> (x^2=w77:dbl[])
      n274 = Add(x=w78, y=w77) -> (x+y=w76:dbl[])
      n275 = Square Root(x=w76) -> (sqrt(x)=w75:dbl[])
      n276 = Bundle(w21, w75) -> (→"uniformity":cluster{i32[], dbl[]})  [unwired: 1 in]
      n277 = case shown="True" "Ins loaded" {
        tunnel: w22 -> [_ _]
        tunnel: w12 -> [w88 w91]
        tunnel: w20 -> [_ _]
        tunnel: w19 -> [w89 w93]
        tunnel: [w89 w92] -> w10
        tunnel: [w88 w90] -> w9
        frame False {
        }
        frame True {
          n278 = call-poly <vilib>:"Read Delimited Spreadsheet.vi"("file path (dialog if empty)"="Psi data base 2") -> ("all rows"=w108:dbl[][])  [unwired: 9 in, 5 out]
          n279 = call-poly <vilib>:"Read Delimited Spreadsheet.vi"("file path (dialog if empty)"="Psi data base 2") -> ("all rows"=w99:dbl[][])  [unwired: 9 in, 5 out]
          n280 = Array Subset(array=w108, index (col)=2 ("index"), length (col)=1 ("length")) -> (w104:dbl[][])  [unwired: 2 in]
          n281 = Array Subset(array=w99, index (col)=3 ("index"), length (col)=1 ("length")) -> (w100:dbl[][])  [unwired: 2 in]
          n282 = Array Size(array=w104) -> (size(s)=w106:i32[])
          n283 = Array Size(array=w100) -> (size(s)=w102:i32[])
          n284 = Array Max & Min(array=w106) -> (max value=w105:i32)  [unwired: 3 out]
          n285 = Array Max & Min(array=w102) -> (max value=w101:i32)  [unwired: 3 out]
          n286 = Reshape Array(w104, w105) -> (w95:dbl[])
          n287 = Reshape Array(w100, w101) -> (w94:dbl[])
          n288 = for {
            tunnel: w91 -> [w122] mode=indexing
            tunnel: [w117] -> w92 mode=indexing
            tunnel: [w109] -> w90 mode=indexing
            tunnel: w95 -> [w115] mode=indexing
            tunnel: w94 -> [w114] mode=indexing
            tunnel: w93 -> [w113] mode=indexing
            n289 = expression code="(x/180.0)*pi" "degrees to radians"(w113) -> (w123:dbl)
            n290 = expression code="(x/180.0)*pi" "degrees to radians"(w122) -> (w121:dbl)
            n291 = expression code="(x/180.0)*pi" "degrees to radians"(w115) -> (w120:dbl)
            n292 = expression code="(x/180.0)*pi" "degrees to radians"(w114) -> (w119:dbl)
            n293 = formula code="float p2,d2;\np2=atan(tan(p1)\n         /tan(p3));\nd2=d1-d3;"("p3"=w120, "d3"=w119, "p1"=w123, "d1"=w121) -> ("p2"=w118:dbl, "d2"=w116:dbl)
            n294 = expression code="(x/pi)*180.0" "radians to degrees"(w118) -> (w117:dbl)
            n295 = expression code="(x/pi)*180.0" "radians to degrees"(w116) -> (w110:dbl)
            n296 = Greater?(x=w110, y=360.0) -> (0:w112:bool)
            n297 = case shown="False" w112 {
              tunnel: w110 -> [w124 w126]
              tunnel: [w124 w125] -> w109
              frame False {
              }
              frame True {
                n298 = Subtract(x=w126, y=360.0) -> (x-y=w125:dbl)
              }
            }
          }
        }
      }
      n299 = Bundle(w21, w22) -> (w13:cluster{i32[], dbl[]})  [unwired: 1 in]
      n300 = Bundle(w21, w20) -> (w25:cluster{i32[], dbl[]})  [unwired: 1 in]
      n301 = Array Subset(array=w37, index (col)=0 ("index"), length (col)=1 ("length")) -> (w39:dbl[][])  [unwired: 2 in]
      n302 = Array Size(array=w39) -> (size(s)=w41:i32[])
      n303 = Array Max & Min(array=w41) -> (max value=w40:i32)  [unwired: 3 out]
      n304 = Reshape Array(w39, w40) -> (w36:dbl[])
      n305 = Bundle(w21, w10) -> (w82:cluster{i32[], dbl[]})  [unwired: 1 in]
      n306 = Bundle(w21, w9) -> (w81:cluster{i32[], dbl[]})  [unwired: 1 in]
      n307 = Bundle(w36, w27) -> (w35:cluster{dbl[], dbl[]})  [unwired: 1 in]
      n308 = Bundle(w36, w26) -> (w34:cluster{dbl[], dbl[]})  [unwired: 1 in]
      n309 = Build Array(w82, w81, w35, w34, w25, w13) -> (→"ALL":cluster{dbl[], dbl[]}[])
      n310 = Tick Count (ms)() -> (millisecond timer value=w86:u32)
    }
    frame #1 {
      n311 = Tick Count (ms)() -> (millisecond timer value=w688:u32)
      n312 = case shown="True" w679 {
        tunnel: w680 -> [_ w720]
        tunnel: w678 -> [_ w717]
        tunnel: w677 -> [_ w716]
        tunnel: w676 -> [_ w715]
        tunnel: w675 -> [_ w694]
        tunnel: w674 -> [_ w695]
        frame False {
        }
        frame True {
          w696 = i8 0
          n313 = local read "x+1"() -> (w707:i8)
          n314 = Increment(x=w707) -> (x+1=w706:i8)
          n315 = for {
            N: w706 -> [_]
            tunnel: [w721] -> w698 mode=indexing
            tunnel: [w721] -> w712
            n316 = case shown="\"65\"" "Angle of Incidence :" {
              tunnel: [i8 25 i8 30 i8 35 i8 40 i8 45 i8 50 i8 55 i8 60 i8 65 i8 70 i8 75 i8 80] -> w721
              frame "25", Default {
              }
              frame "30" {
              }
              frame "35" {
              }
              frame "40" {
              }
              frame "45" {
              }
              frame "50" {
              }
              frame "55" {
              }
              frame "60" {
              }
              frame "65" {
              }
              frame "70" {
              }
              frame "75" {
              }
              frame "80" {
              }
            }
          }
          n317 = Build Array (concatenate)(w696, w716) -> (w713:dbl[])
          n318 = Build Array (concatenate)(w696, w715) -> (w714:dbl[])
          n319 = Build Array (concatenate)(w696, w717) -> (w697:i32[])
          n320 = Build Array (concatenate)(w696, w695) -> (w693:dbl[])
          n321 = Build Array (concatenate)(w696, w694) -> (w692:dbl[])
          n322 = Number To Decimal String(number=w712) -> (decimal integer string=w710:string)  [unwired: 1 in]
          n323 = Build Array(w697, w698, w713, w714) -> (w718:dbl[][])
          n324 = Build Array(w697, w698, w693, w692) -> (w702:dbl[][])
          n325 = Transpose 2D Array(2D array=w718) -> (transposed array=w705:dbl[][])
          n326 = Transpose 2D Array(2D array=w702) -> (transposed array=w701:dbl[][])
          "transposed array" <- w701
          n327 = Array Subset(array=w701, index (row)=1 ("index")) -> (w699:dbl[][])  [unwired: 3 in]
          n328 = Concatenate Strings("AOI_" ("String"), w710, "_SE data" ("String")) -> (w708:string)
          n329 = Array Subset(array=w705, index (row)=1 ("index")) -> (w703:dbl[][])  [unwired: 3 in]
          n330 = case shown="True" "SE BMP & Txt File" {
            tunnel: w708 -> [_ w742]
            tunnel: w703 -> [_ w768]
            tunnel: w720 -> [_ w763]
            tunnel: w699 -> [_ w743]
            frame False {
            }
            frame True {
              w752 = ".bmp" ("string")
              n331 = Strip Path(path=w763) -> (stripped path=w761:path)  [unwired: 1 out]
              n332 = Concatenate Strings(w742) -> (w740:string)
              n333 = Concatenate Strings(w742, ".txt" ("string")) -> (w776:string)
              n334 = Build Path(base path=w761, name or relative path=w742) -> (appended path=w764:path)
              n335 = String To Path(string=w740) -> (path=w739:path)
              n336 = call <vilib>:"Check if File or Folder Exists.vi"("path"=w764) -> ("file or folder exists?"=w765:bool, "dup path"=w766:path)  [unwired: 8 in, 1 out]
              n337 = Concatenate Strings(w742, "_Ins_polar.txt" ("string")) -> (w744:string)
              n338 = case shown="False" w765 {
                tunnel: w766 -> [w780 w783]
                tunnel: [w779 w782] -> w741
                tunnel: w742 -> [w777 w781]
                frame False {
                  n339 = Create Folder(path (use dialog)=w780) -> (created path=w778:path)  [unwired: 2 in, 2 out]
                  n340 = Build Path(base path=w778, name or relative path=w777) -> (appended path=w779:path)
                }
                frame True {
                  n341 = Build Path(base path=w783, name or relative path=w781) -> (appended path=w782:path)
                }
              }
              n342 = Path To String(path=w741) -> (string=w759:string)
              n343 = Path To String(path=w741) -> (string=w762:string)
              n344 = Concatenate Strings(w752) -> (w758:string)
              n345 = Build Path(base path=w741, name or relative path=w739) -> (appended path=w736:path)
              n346 = Concatenate Strings("ROI" ("string"), w752) -> ()  [unwired: 1 out]
              n347 = Concatenate Strings(w759, w758) -> (w760:string)
              n348 = Concatenate Strings(w762, w742) -> (w775:string)
              n349 = Strip Path(path=w736) -> (stripped path=w735:path)  [unwired: 1 out]
              n350 = String To Path(string=w760) -> (path=w753:path)
              n351 = String To Path(string=w775) -> (path=w746:path)
              n352 = call-poly <vilib>:"Write Delimited Spreadsheet.vi"("file path (dialog if empty)"=w735, "2D data"=w743, "append to file? (new file:F)"=FALSE) -> ("new file path (Not A Path if cancelled)"=w737:path)  [unwired: 11 in, 1 out]
              n353 = Strip Path(path=w737) -> (stripped path=w738:path)  [unwired: 1 out]
              n354 = call-poly <vilib>:"Write Delimited Spreadsheet.vi"("file path (dialog if empty)"=w746, "2D data"=w768, "append to file? (new file:F)"=FALSE) -> ("new file path (Not A Path if cancelled)"=w769:path)  [unwired: 11 in, 1 out]
              n355 = invoke on="ALL" class="XYGraph (strict)" method="Export Image"("FileType"=enum32{"BMP", "EPS", "EMF", "PICT"}."BMP" ("File Type"), "Target"=enum32{"File", "Clipboard"}."File", "Path"=w753, "HideGrid"=TRUE ("Hide Grid"), "Overwrite"=TRUE ("Always Overwrite")) -> ()  [unwired: 3 in, 8 out]
              n356 = Strip Path(path=w769) -> (stripped path=w773:path)  [unwired: 1 out]
              n357 = Build Path(base path=w738, name or relative path=w744) -> (appended path=w749:path)
              n358 = Build Path(base path=w773, name or relative path=w776) -> (appended path=w772:path)
              n359 = Copy(9:TRUE ("overwrite (F)"), 10:w749, 11:w737) -> (0:w750:errorcluster)  [unwired: 2 in, 2 out]
              n360 = Delete(path (use dialog)=w737, error in=w750) -> ()  [unwired: 3 in, 3 out]
              n361 = Copy(9:TRUE ("overwrite (F)"), 10:w772, 11:w769) -> (0:w774:errorcluster)  [unwired: 2 in, 2 out]
              n362 = Delete(path (use dialog)=w769, error in=w774) -> ()  [unwired: 3 in, 3 out]
            }
          }
        }
      }
      n363 = Subtract(x=w688, y=w681) -> (x-y=w689:u32)
      n364 = Divide(x=w689, y=u32 1000) -> (x/y=w690:dbl)
      n365 = Quotient & Remainder(x=w690, y=60.0) -> (x-y*floor(x/y)=→"Seconds":dbl, floor(x/y)=w691:dbl)
      n366 = Quotient & Remainder(x=w691, y=60.0) -> (x-y*floor(x/y)=→"Minutes":dbl, floor(x/y)=→"Hours":dbl)
    }
  }
